vi "OFDM_Demodulation.vi"(9 "sampling period":dbl format="%#_13g", 10 "Frequency channel estimation":cdb[](array[numeric]) format="%.2f", 11 "Input sequence":cdb[](array[numeric])) -> (3 "Output sequence":cdb[](array[numeric]))   [LabVIEW 2018]
uses:
  <vilib>/Analysis/2dsp.llb/Complex FFT.vi
  <vilib>/Analysis/baseanly.llb/Mean (CDB).vi
  <vilib>/Analysis/NI_AALPro.lvlib
  <vilib>/Analysis/NI_AALBase.lvlib
panel:
  out "x/y":cdb[](array[numeric])
  out "Waveform Graph":dbl[](graph)
  out "size(s)":i32
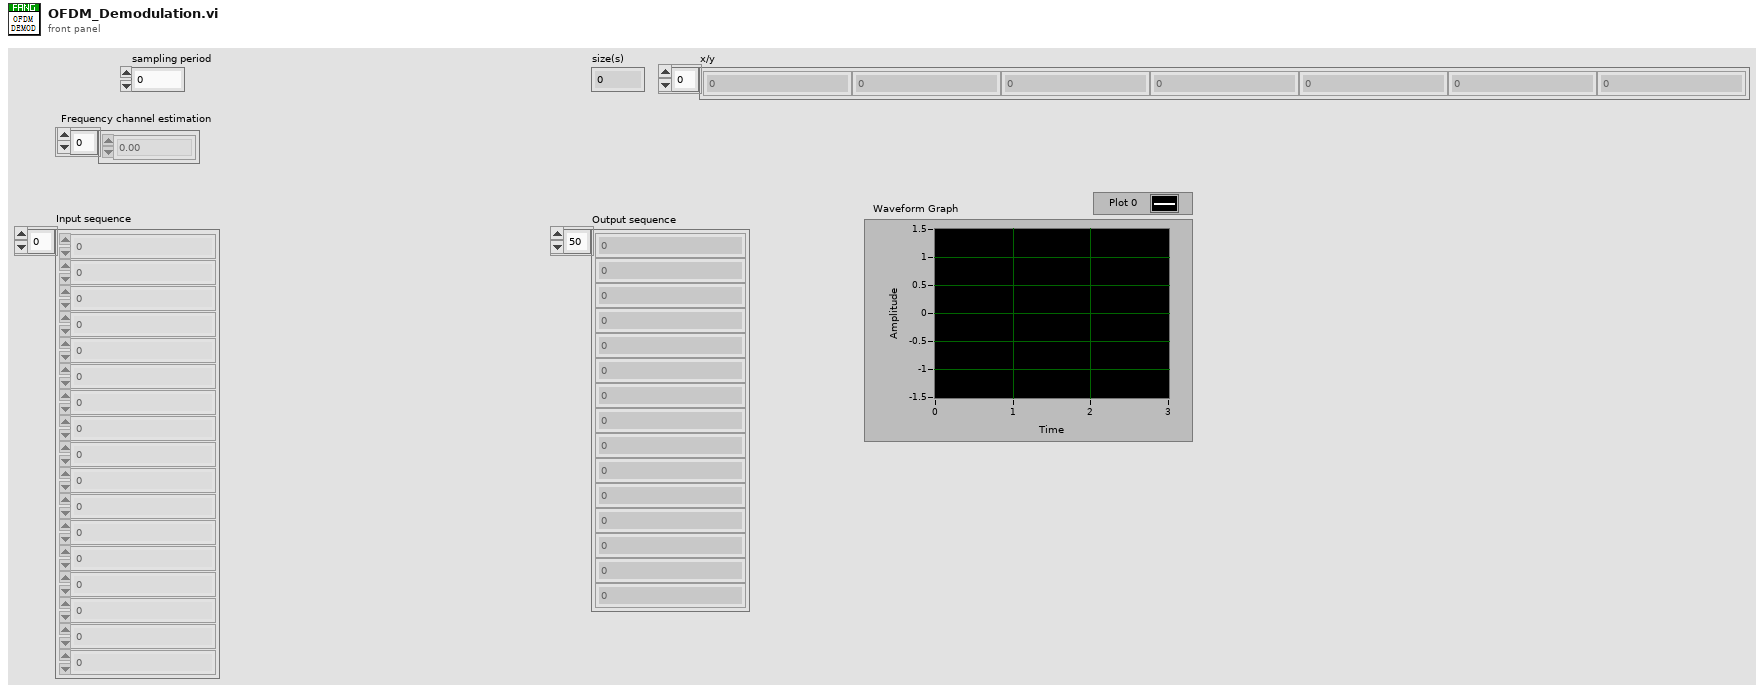
[diagram p1: front panel]
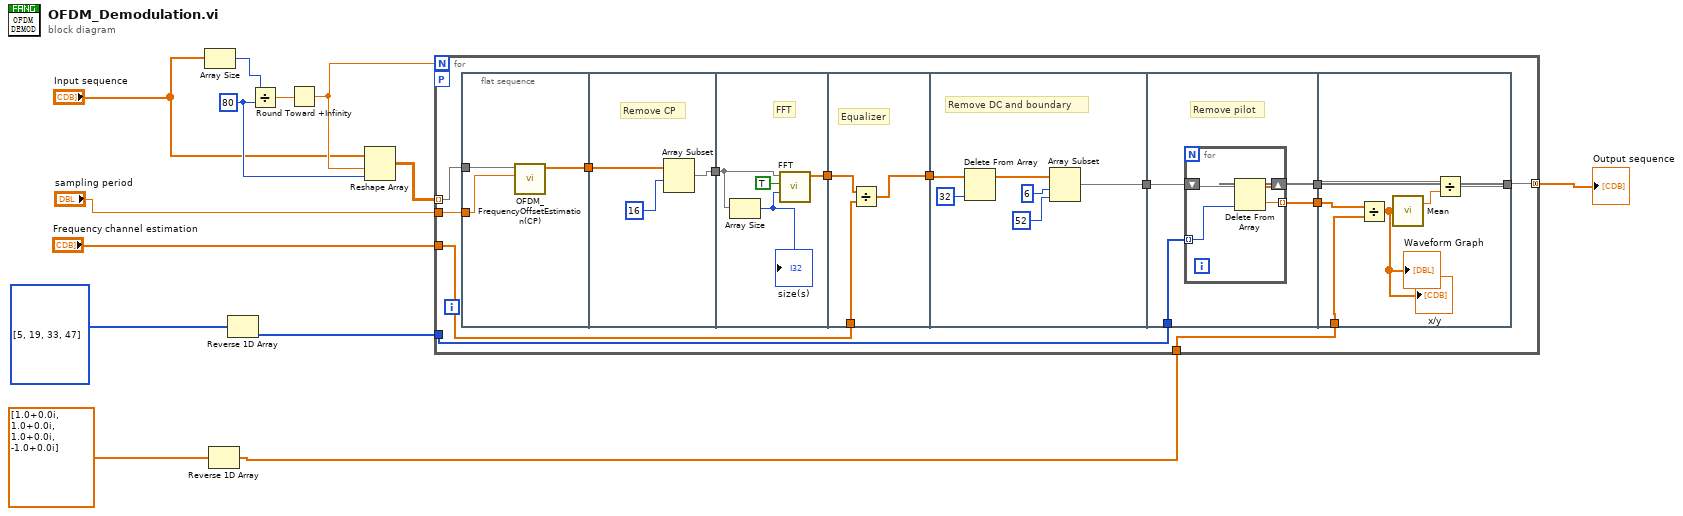
[diagram p0: block diagram]
diagram:
  w9 = 80 ("y")
  n1 = Array Size(array="Input sequence") -> (size(s)=w13:i32)
  n2 = Reverse 1D Array(array=cdb[] [1.0+0.0i, 1.0+0.0i, 1.0+0.0i, -1.0+0.0i]) -> (reversed array=w2:cdb[])
  n3 = Reverse 1D Array(array=i32[] [5, 19, 33, 47]) -> (reversed array=w7:i32[])
  n4 = Divide(x=w13, y=w9) -> (x/y=w12:dbl)
  n5 = Round Toward +Infinity(x=w12) -> (ceil(x): smallest int >= x=w10:dbl)
  n6 = Reshape Array("Input sequence", w10, w9) -> (w11:cdb[][])
  n7 = for {
    N: w10 -> [_]
    tunnel: w11 -> [w24] mode=indexing
    tunnel: w7 -> [w25]
    tunnel: [w19] -> w6 mode=concatenating
    tunnel: "Frequency channel estimation" -> [w21]
    tunnel: w2 -> [w16]
    workers-P: _ -> [_]
    tunnel: "sampling period" -> [w14]
    n8 = flat-sequence {
      tunnel: w24 -> [w29]
      tunnel: [w28] -> w15
      tunnel: w14 -> [w27]
      tunnel: [w30] -> w22
      tunnel: w15 -> [w32]
      tunnel: [w34] -> w23
      tunnel: w22 -> [w33]
      tunnel: w23 -> [w38]
      tunnel: w21 -> [w39]
      tunnel: [w37] -> w20
      tunnel: [w40] -> w26
      tunnel: w20 -> [w43]
      tunnel: w26 -> [w49]
      tunnel: w25 -> [w48]
      tunnel: [w47] -> w18
      tunnel: [w46] -> w17
      tunnel: [w56] -> w19
      tunnel: w18 -> [w57]
      tunnel: w17 -> [w55]
      tunnel: w16 -> [w59]
      frame #0 {
        n9 = call "OFDM_FrequencyOffsetEstimation(CP).vi"("sampling period"=w27, "input OFDM symbol"=w29) -> ("output OFDM symbol"=w28:cdb[])  [unwired: 9 in]
      }
      frame #1 {
        # "Remove CP"
        n10 = Array Subset(array=w32, index=16) -> (w30:cdb[])  [unwired: 1 in]
      }
      frame #2 {
        # "FFT"
        n11 = Array Size(array=w33) -> (size(s)=w35:i32)
        "size(s)" <- w35
        n12 = call-poly <vilib>:"FFT.vi"("FFT size"=w35, "shift?"=TRUE, "X"=w33) -> ("FFT {X}"=w34:cdb[])  [unwired: 7 in, 1 out]
      }
      frame #3 {
        # "Equalizer"
        n13 = Divide(x=w38, y=w39) -> (x/y=w37:cdb[])
      }
      frame #4 {
        # "Remove DC and boundary"
        n14 = Delete From Array(array=w43, index=32) -> (array with subset deleted=w41:cdb[])  [unwired: 1 in, 1 out]
        n15 = Array Subset(array=w41, index=6, length=52) -> (w40:cdb[])
      }
      frame #5 {
        # "Remove pilot"
        n16 = for {
          shift-right: [w53] -> w47
          shift-left: w49 -> [w52]
          tunnel: w48 -> [w51] mode=indexing
          tunnel: [w50] -> w46 mode=indexing
          n17 = Delete From Array(array=w52, index=w51) -> (deleted portion=w50:cdb, array with subset deleted=w53:cdb[])  [unwired: 1 in]
        }
      }
      frame #6 {
        n18 = Divide(x=w55, y=w59) -> (x/y=w54:cdb[])
        "Waveform Graph" <- w54
        "x/y" <- w54
        n19 = call-poly <vilib>:"Mean.vi"("X"=w54) -> ("mean"=w58:cdb)  [unwired: 1 out]
        n20 = Divide(x=w57, y=w58) -> (x/y=w56:cdb[])
      }
    }
  }
  "Output sequence" <- w6
